vi "BuildVI.vi"(8 "error in (no error)":errorcluster, 10 "Name":string, 11 "CreateInterface in":refnum<class "CreateInterface.lvclass">) -> (0 "error out":errorcluster, 3 "CreateInterface out":refnum<class "CreateInterface.lvclass">)   [LabVIEW 2020, in "Mermaid.lvlib" / "CreateInterface.lvclass"]
uses:
  CreateInterface.lvclass
  CreateInterface.lvclass/CreateInterface.ctl
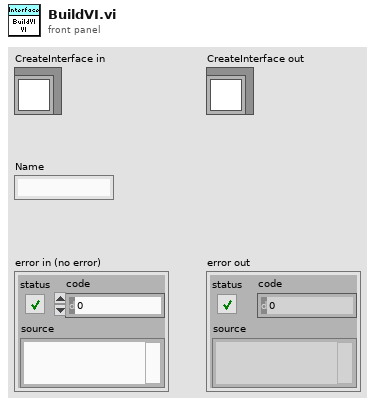
[diagram p1: front panel]
types:
  T1 = enum32{"invalid VI type", "Standard VI", "Control VI", "Global VI", "Polymorphic VI", "Configuration VI", "SubSystem", "Facade VI", "Method VI", "Statechart Diagram VI"}
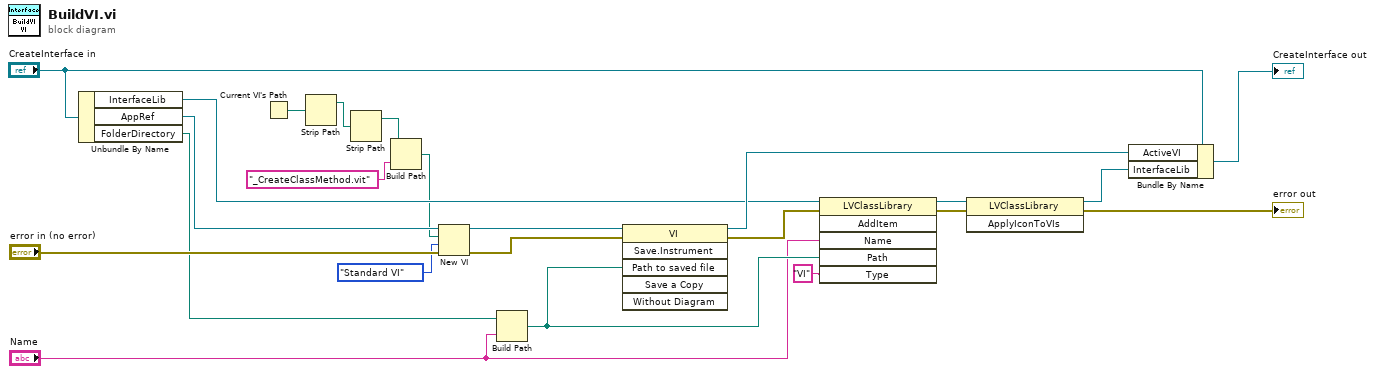
[diagram p0: block diagram]
diagram:
  n1 = Unbundle By Name("CreateInterface in") -> ("InterfaceLib"=w18:refnum<vi>, "AppRef"=w17:refnum<vi>, "FolderDirectory"=w6:path)
  n2 = Current VI's Path() -> (path=w5:path)
  n3 = Strip Path(path=w5) -> (stripped path=w2:path)  [unwired: 1 out]
  n4 = Strip Path(path=w2) -> (stripped path=w3:path)  [unwired: 1 out]
  n5 = Build Path(base path=w3, name or relative path="_CreateClassMethod.vit" ("Name")) -> (appended path=w4:path)
  n6 = New VI(8:"error in (no error)", 9:T1."Standard VI" ("vi type (standard vi)"), 10:w4, 11:w17) -> (0:w8:errorcluster, 3:w7:refnum<vi>)  [unwired: 3 in]
  n7 = Build Path(base path=w6, name or relative path="Name") -> (appended path=w10:path)
  n8 = invoke class="VI" method="Save.Instrument"(reference=w7, error in=w8, "Path to saved file"=w10) -> (reference out=w19:refnum<vi>, error out=w9:errorcluster)  [unwired: 3 in, 4 out]
  n9 = invoke class="LVClassLibrary" method="AddItem"(reference=w18, error in=w9, "Name"="Name", "Path"=w10, "Type"="VI") -> (reference out=w14:refnum<vi>, error out=w15:errorcluster)  [unwired: 1 in, 4 out]
  n10 = invoke class="LVClassLibrary" method="ApplyIconToVIs"(reference=w14, error in=w15) -> (reference out=w23:refnum<vi>, error out=→"error out":errorcluster)  [unwired: 1 in, 1 out]
  n11 = Bundle By Name(cluster="CreateInterface in", "ActiveVI"=w19, "InterfaceLib"=w23) -> (→"CreateInterface out":refnum<class "CreateInterface.lvclass">)
